vi "ConvectronSerial.vi"() -> ()   [LabVIEW 2019]
doc: "This example performs a serial port write and a serial port read. The parameters set for the serial port must match the parameters of the connected instrument or device. The VISA Configure Serial Port VI sets the configuration parameters. The front panel displays the controls used to configure the basic parameters, such as baud rate, data bits, and parity. The VI passes the VISA resource name to other VIs that perform operations on that VISA resource. The VISA Write function sends a command to the serial device and the VISA Read function returns data based on the command. The VISA Close function then closes the reference to the serial device. It is important to close the reference; otherwise, further communication through that port might not be possible."
uses:
  Program Files/National Instruments/LabVIEW 2019/examples/Instrument IO/Serial/support/Serial - Settings.ctl
  <vilib>/Instr/_visa.llb/VISA Configure Serial Port (Instr).vi
  <vilib>/Utility/file.llb/Read Delimited Spreadsheet (DBL).vi
  <vilib>/gmath/NI_Gmath.lvlib
panel:
  in  "Gas Type":u16(ring)=1 items=["Air", "Krypton"]
  in  "Lookup Table File":path=path "C:/Users/jfrechem/Box/Frechem Dissertation - Working Folder/Research Files/Convectron Calibration/KryptonTranspose.csv"
  out "Convectron":waveform(dbl)(graph)={"t0"=timestamp(3663606467.378807 s since 1904-01-01), "dt"=1.0, "Y"=[0.21643555984555984]}
  in  "Filename":path=path "C:/Users/jfrechem/Desktop/200mTorr_Overnight.xlsx"
  in  "Write to file":bool caption="Enable"
  in  "stop":bool
  out "Pressure":dbl=0.21643555984555984 format="%#_3e"
  in  "Serial Settings":T1={"baud rate"=19200, "data bits"=8, "parity"=enum."None", "stop bits"=10, "flow control"=2} {"flow control" items=["None"=0, "XON/XOFF"=1, "RTS/CTS"=2, "DTR/DSR"=4]; "stop bits" items=["1.0"=10, "1.5"=15, "2.0"=20]; "data bits" min=5 max=8 step=1; "baud rate" items=["75"=75, "110"=110, "134"=134, "150"=150, "300"=300, "600"=600, "1200"=1200, "1800"=1800, "2400"=2400, "4800"=4800, "7200"=7200, "9600"=9600, "14400"=14400, "19200"=19200, "28800"=28800, "38400"=38400, "56000"=56000, "57600"=57600, "115200"=115200, "128000"=128000, "230400"=230400]}
  in  "Read Period (s)":dbl=1.0
  out "Response":string="9.92E-02\r"
  in  "VISA resource name":refnum<visa-resource-name>="COM1"
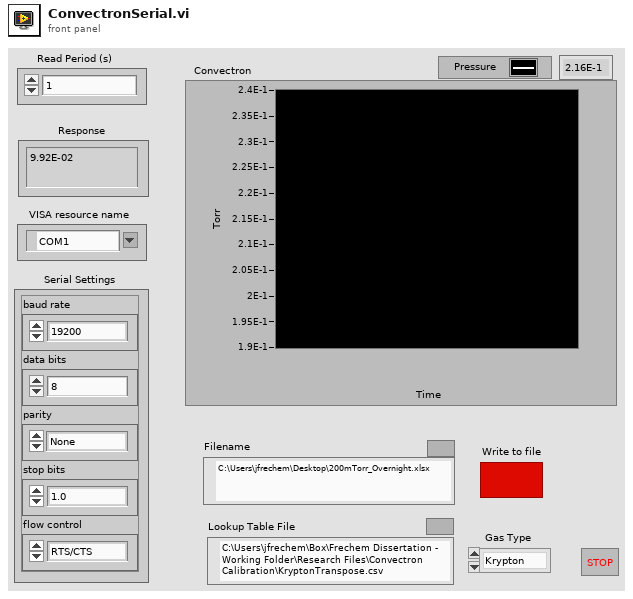
[diagram p1: front panel]
types:
  T1 = typedef "Serial - Settings.ctl" = cluster{"baud rate":u32, "data bits":u16, "parity":enum16{"None", "Odd", "Even", "Mark", "Space"}, "stop bits":u16, "flow control":u16}
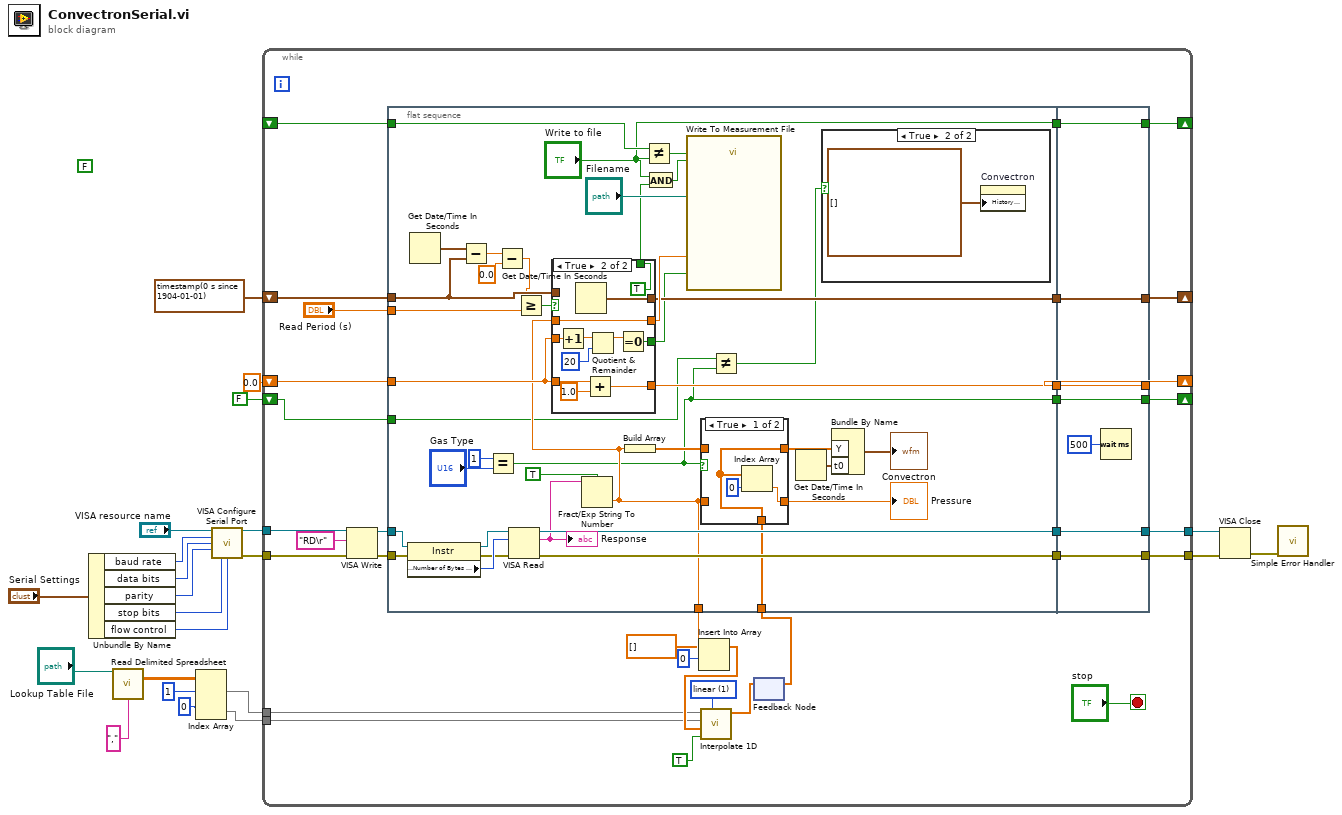
[diagram p0: block diagram]
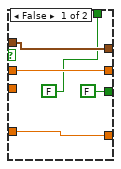
[diagram p4: hidden frame]
diagram:
  (unwired) FALSE
  n1 = Unbundle By Name("Serial Settings") -> ("baud rate"=w18:u32, "data bits"=w17:u16, "parity"=w16:enum16{"None", "Odd", "Even", "Mark", "Space"}, "stop bits"=w15:u16, "flow control"=w14:u16)
  n2 = call-poly <vilib>:"Read Delimited Spreadsheet.vi"("file path (dialog if empty)"="Lookup Table File", "delimiter (\\t)"="," ("delimiter (\\t)")) -> ("all rows"=w6:dbl[][])  [unwired: 8 in, 5 out]
  n3 = Index Array(array=w6, index (row) #1=1 ("index (row)"), index (row) #2=0 ("index (row)")) -> (element #1=w3:dbl[], element #2=w2:dbl[])  [unwired: 2 in]
  n4 = call-poly "VISA Configure Serial Port"("VISA resource name"="VISA resource name", "baud rate (9600)"=w18, "data bits (8)"=w17, "parity (0:none)"=w16, "stop bits (10: 1 bit)"=w15, "flow control (0:none)"=w14) -> ("VISA resource name out"=w20:refnum<visa-resource-name>, "error out"=w21:errorcluster)  [unwired: 3 in, 5 out]
  n5 = while {
    tunnel: w20 -> [w54]
    tunnel: w21 -> [w55]
    tunnel: [w52] -> w12
    tunnel: [w51] -> w11
    shift-right: [w45] -> _
    shift-left: timestamp(0 s since 1904-01-01) ("seconds since 1Jan1904") -> [w43]
    shift-right: [w39] -> _
    shift-left: 0.0 -> [w41]
    shift-right: [w37] -> _
    shift-left: _ -> [w36]
    tunnel: w2 -> [w28]
    tunnel: w3 -> [w29]
    shift-right: [w24] -> _
    shift-left: FALSE -> [w23]
    stop <- "stop" stop-if-true
    w30 = 1 items=["nearest", "linear", "spline", "cubic Hermite", "Lagrange"] ("method")
    n6 = VISA Write(VISA resource name=w54, write buffer="RD\r" ("Command"), error in (no error)=w55) -> (VISA resource name out=w48:refnum<visa-resource-name>, error out=w47:errorcluster)  [unwired: 1 out]
    n7 = flat-sequence {
      tunnel: w48 -> [w91]
      tunnel: w47 -> [w90]
      tunnel: [w89] -> w50
      tunnel: [w88] -> w49
      tunnel: [w81] -> w44
      tunnel: w43 -> [w78]
      tunnel: "Read Period (s)" -> [w76]
      tunnel: w41 -> [w74]
      tunnel: [w75] -> w40
      tunnel: ["Write to file"] -> w38
      tunnel: w36 -> [w70]
      tunnel: [w64] -> w33
      tunnel: w27 -> [w61]
      tunnel: [w57] -> w25
      tunnel: w23 -> [w58]
      tunnel: [w122] -> w51
      tunnel: [w123] -> w52
      tunnel: w50 -> [w123]
      tunnel: w49 -> [w122]
      tunnel: [w121] -> w45
      tunnel: w44 -> [w121]
      tunnel: [w119] -> w39
      tunnel: w40 -> [w119]
      tunnel: [w118] -> w37
      tunnel: w38 -> [w118]
      tunnel: [w117] -> w24
      tunnel: w25 -> [w117]
      frame #0 {
        n8 = property class="Instr"(reference=w91, error in=w90) -> (reference out=w92:refnum<visa-resource-name>, error out=w93:errorcluster, "Serial Settings:Number of Bytes at Serial Port"=w94:u32)
        n9 = Get Date/Time In Seconds() -> (seconds since 1Jan1904=w79:timestamp)
        n10 = Subtract(x=w79, y=w78) -> (x-y=w68:dbl)
        n11 = Equal?(x=u16 1, y="Gas Type") -> (x = y?=w57:bool)
        n12 = Subtract(x=w68, y=0.0) -> (x-y=w67:dbl)
        n13 = VISA Read(VISA resource name=w92, byte count=w94, error in (no error)=w93) -> (VISA resource name out=w88:refnum<visa-resource-name>, read buffer=w87:string, error out=w89:errorcluster)  [unwired: 1 out]
        "Response" <- w87
        n14 = Greater Or Equal?(x=w67, y=w76) -> (x >= y?=w80:bool)
        n15 = Fract/Exp String To Number(use system decimal point (T)=TRUE, string=w87) -> (number=w64:dbl)  [unwired: 2 in, 1 out]
        n16 = case shown="True" w80 {
          tunnel: w64 -> [w102 w116]
          tunnel: [w102 w116] -> w82
          tunnel: [w105 w115] -> w81
          tunnel: w78 -> [w105 _]
          tunnel: [FALSE w111] -> w77
          tunnel: [w103 w110] -> w75
          tunnel: w74 -> [w103 w108]
          tunnel: w74 -> [_ w107]
          tunnel: [FALSE TRUE] -> w73
          frame False {
          }
          frame True {
            n17 = Increment(x=w107) -> (x+1=w114:dbl)
            n18 = Get Date/Time In Seconds() -> (seconds since 1Jan1904=w115:timestamp)
            n19 = Add(x=w108, y=1.0) -> (x+y=w110:dbl)
            n20 = Quotient & Remainder(x=w114, y=20) -> (x-y*floor(x/y)=w112:dbl)  [unwired: 1 out]
            n21 = Equal To 0?(x=w112) -> (x = 0?=w111:bool)
          }
        }
        n22 = Build Array(w64) -> (w63:dbl[])
        n23 = Not Equal?(x=w70, y="Write to file") -> (x != y?=w71:bool)
        n24 = And(x="Write to file", y=w73) -> (x .and. y?=w72:bool)
        n25 = call "Write To Measurement File"("Signals"=w82, "Reset"=w71, "Enable"=w72, "Flush? (T)"=w77, "Filename"="Filename") -> ()  [unwired: 12 in, 3 out]
        n26 = case shown="True" w57 {
          tunnel: [w98 w100] -> w65
          tunnel: w64 -> [_ w100]
          tunnel: w63 -> [_ w99]
          tunnel: [w97 w99] -> w62
          tunnel: w61 -> [w97 _]
          frame True {
            n27 = Index Array(array=w97, index=0) -> (element=w98:dbl)
          }
          frame False {
          }
        }
        "Pressure" <- w65
        n28 = Not Equal?(x=w58, y=w57) -> (x != y?=w56:bool)
        n29 = Get Date/Time In Seconds() -> (seconds since 1Jan1904=w84:timestamp)
        n30 = case shown="True" w56 {
          frame False {
          }
          frame True {
            n31 = property on="Convectron" class="WFChart (strict)"("History Data"=waveform(dbl)[] []) -> ()  [unwired: 2 in, 2 out]
          }
        }
        n32 = Bundle By Name("Y"=w62, "t0"=w84) -> (→"Convectron":waveform(dbl))  [unwired: 1 in]
      }
      frame #1 {
        n33 = Wait (ms)(milliseconds to wait=u32 500) -> ()  [unwired: 1 out]
      }
    }
    n34 = Insert Into Array(array=dbl[] [], index=0, new element=w33) -> (w32:dbl[])
    n35 = call <vilib>:"Interpolate 1D.vi"("method"=w30, "X is monotonic"=TRUE, "xi"=w32, "X"=w28, "Y"=w29) -> ("yi"=w26:dbl[])  [unwired: 4 in, 2 out]
    n36 = feedback-in #1(w26) -> ()
    n37 = feedback #1() -> (w27:dbl[])  [unwired: 1 in]
  }
  n38 = VISA Close(VISA resource name=w11, error in (no error)=w12) -> (error out=w13:errorcluster)
  n39 = call <vilib>:"Simple Error Handler.vi"("error in (no error)"=w13) -> ()  [unwired: 1 in, 8 out]
